vi "removeLink.vi"(8 "error in (no error)":errorcluster, 10 "subNode in":refnum<data-value>, 11 "superNode in":refnum<class "xceNode.lvclass">) -> (0 "error out":errorcluster, 2 "subNode out":refnum<data-value>, 3 "superNode out":refnum<class "xceNode.lvclass">)   [LabVIEW 2013, in "xceNode.lvclass"]
doc: "Removes a link between a subNode and a superNode. Used to remove a node from the tree data structure, or drag a node to a different location."
uses:
  xceNode.lvclass
  xceNode.lvclass/xceNode.ctl
  xceTreeObj/xceTreeObj.lvclass
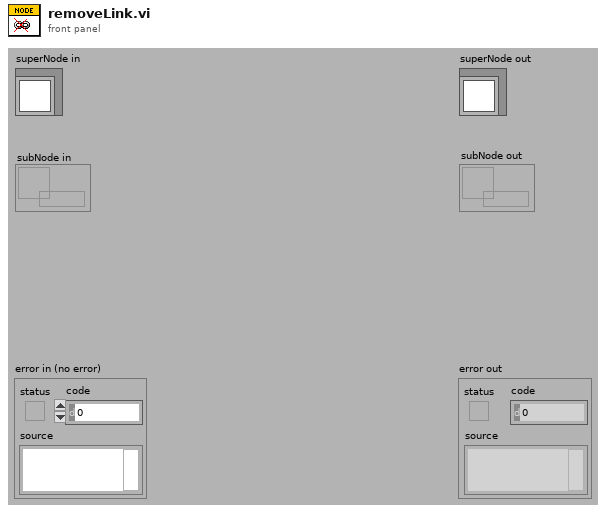
[diagram p1: front panel]
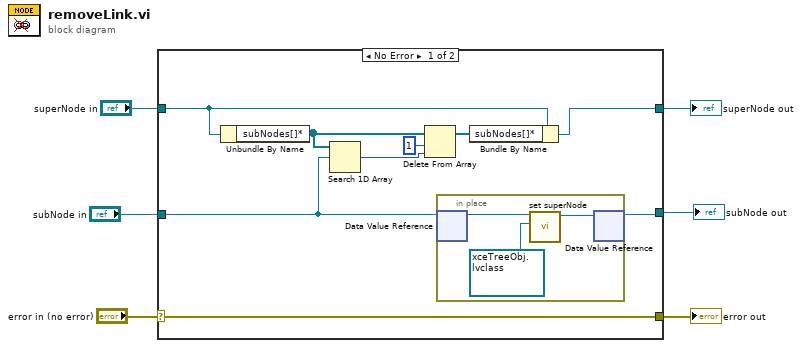
[diagram p0: block diagram]
diagram:
  n1 = case shown="No Error" "error in (no error)" {
    selector: "error in (no error)" -> [w15 w20]
    tunnel: [w15 w20] -> w5
    tunnel: [w9 w19] -> w3
    tunnel: "superNode in" -> [w11 w19]
    tunnel: "subNode in" -> [w8 _]
    tunnel: [w7 _] -> w1
    frame No Error {
      n2 = Unbundle By Name(w11) -> ("subNodes[]*"=w14:refnum<data-value>[])
      n3 = Search 1D Array(1D array=w14, element=w8) -> (index of element=w13:i32)  [unwired: 1 in]
      n4 = Delete From Array(array=w14, length=1, index=w13) -> (array with subset deleted=w10:refnum<data-value>[])  [unwired: 1 out]
      n5 = in-place {
        n6 = in-place-dvr #1(w8) -> (w18:refnum<class "xceNode.lvclass">)  [unwired: 1 out]
        n7 = call "set superNode.vi"("superNode*"=refnum<data-value> refnum, "xceNode in"=w18) -> ("xceNode out"=w17:refnum<class "xceNode.lvclass">)  [unwired: 8 in, 1 out]
        n8 = in-place-dvr #1(w17) -> (w7:refnum<data-value>)  [unwired: 1 out]
      }
      n9 = Bundle By Name(cluster=w11, "subNodes[]*"=w10) -> (w9:refnum<class "xceNode.lvclass">)
    }
    frame Error {
    }
  }
  "error out" <- w5
  "superNode out" <- w3
  "subNode out" <- w1
